vi "robot_choose_step.vi"(8 "error In":errorcluster, 9 "JSON string":string, 10 "Step order":string, 11 "process_ID":string) -> (0 "error IO":errorcluster)   [LabVIEW 2020]
uses:
  status/filter_vial_No.vi
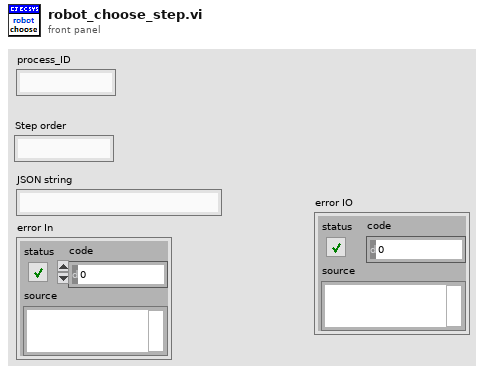
[diagram p1: front panel]
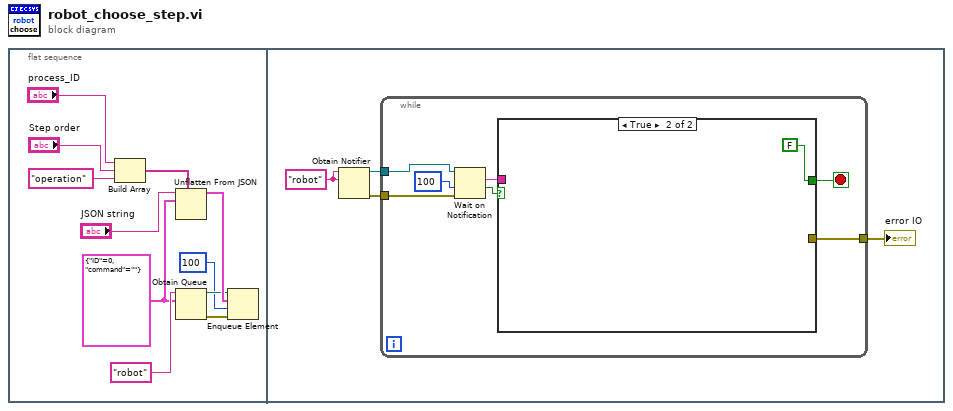
[diagram p0: block diagram]
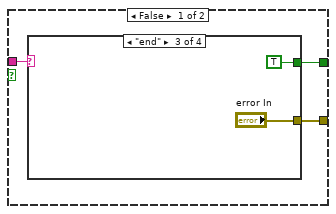
[diagram p2: hidden frame]
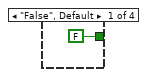
[diagram p3: hidden frame]
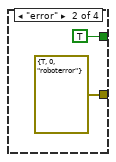
[diagram p4: hidden frame]
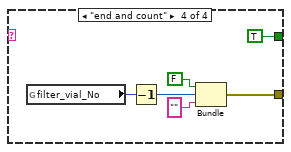
[diagram p5: hidden frame]
diagram:
  n1 = flat-sequence {
    frame #0 {
      w1 = cluster{"ID":i32, "command":string} {"ID"=0, "command"=""} ("参数")
      n2 = Build Array("process_ID", "Step order", "operation" ("string")) -> (w8:string[])
      n3 = Unflatten From JSON(path=w8, JSON string="JSON string", type and defaults=w1) -> (value=w11:cluster{"ID":i32, "command":string})  [unwired: 4 in, 1 out]
      n4 = Obtain Queue(name (unnamed)="robot", element data type=w1) -> (queue out=w9:refnum<queue>, error out=w10:errorcluster)  [unwired: 3 in, 1 out]
      n5 = Enqueue Element(queue=w9, element=w11, timeout in ms (-1)=100, error in (no error)=w10) -> ()  [unwired: 3 out]
    }
    frame #1 {
      w12 = "robot" ("name (unnamed)")
      n6 = Obtain Notifier(name (unnamed)=w12, notification data type=w12) -> (notifier out=w15:refnum<notifier>, error out=w14:errorcluster)  [unwired: 2 in, 1 out]
      n7 = while {
        tunnel: w15 -> [w22]
        tunnel: w14 -> [w19]
        tunnel: [w16] -> w13
        stop <- w17 stop-if-true
        n8 = Wait on Notification(notifier=w22, timeout in ms (-1)=100, error in (no error)=w19) -> (notification=w18:string, timed out?=w20:bool)  [unwired: 1 in, 2 out]
        n9 = case shown="True" w20 {
          tunnel: w18 -> [w23 _]
          tunnel: [w25 FALSE] -> w17
          tunnel: [w24 _] -> w16
          frame False {
            n10 = case shown="\"end\"" w23 {
              tunnel: [FALSE TRUE TRUE TRUE] -> w25
              tunnel: [_ errorcluster {"status"=TRUE, "code"=0, "source"="roboterror"} ("error IO") "error In" w31] -> w24
              frame "False", Default {
              }
              frame "error" {
              }
              frame "end" {
              }
              frame "end and count" {
                n11 = global read "filter_vial_No.vi" "filter_vial_No"() -> (w34:i32)
                n12 = Decrement(x=w34) -> (x-1=w35:i32)
                n13 = Bundle("status"=FALSE, w35, "source"="") -> (w31:cluster{"status":bool, i32, "source":string})  [unwired: 1 in]
              }
            }
          }
          frame True {
          }
        }
      }
      "error IO" <- w13
    }
  }
